vi "Chroma 1905x Series Initialize.vi"(7 "Serial Configuration":T1={"Baud Rate"=9600, "Flow Control"=0, "Parity"=0, "Data Bits"=8, "Stop Bits"=1} {"Flow Control" items=["NONE", "SOFTWARE"]; "Stop Bits" items=["1"=1]; "Data Bits" items=["7"=7, "8"=8]; "Parity" items=["NONE", "ODD", "EVEN"]; "Baud Rate" items=["300"=300, "600"=600, "1200"=1200, "2400"=2400, "4800"=4800, "9600"=9600, "19200"=19200]}, 8 "error in (no error)":errorcluster, 9 "Reset (True)":bool=TRUE, 10 "ID Query (True)":bool=TRUE, 11 "VISA resource name":refnum<visa-resource-name>) -> (0 "error out":errorcluster, 3 "VISA resource name out":refnum<visa-resource-name>)   [LabVIEW 2025]
doc: "This VI passes the addressing information in the instrument decriptor to the Instr Open VI and returns the instrument ID. You can optionally reset the instrument by setting the front panel reset control. You must run this VI before using any of the instrument driver VIs for this instrument."
uses:
  <vilib>/ErrorRing/Error Ring.xnode
  <instrlib>/_Template - Generic/Template - Generic.lvlib
panel:
  # "true\n\nfalse"
  # "true\n\nfalse"
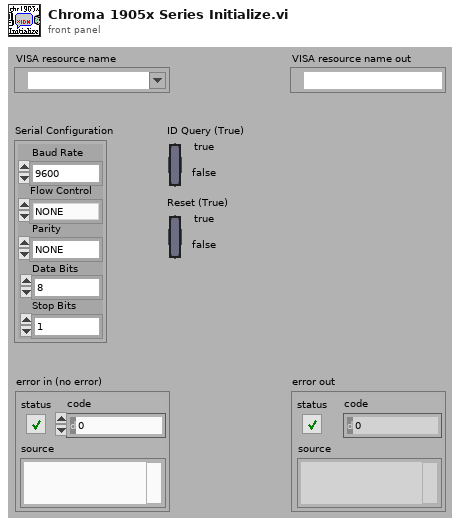
[diagram p1: front panel]
types:
  T1 = cluster{"Baud Rate":u32, "Flow Control":u16, "Parity":u16, "Data Bits":u16, "Stop Bits":u16}
  T2 = cluster{"resource name":string, "interface type":bool, "VISA resource name":refnum<visa-resource-name>}
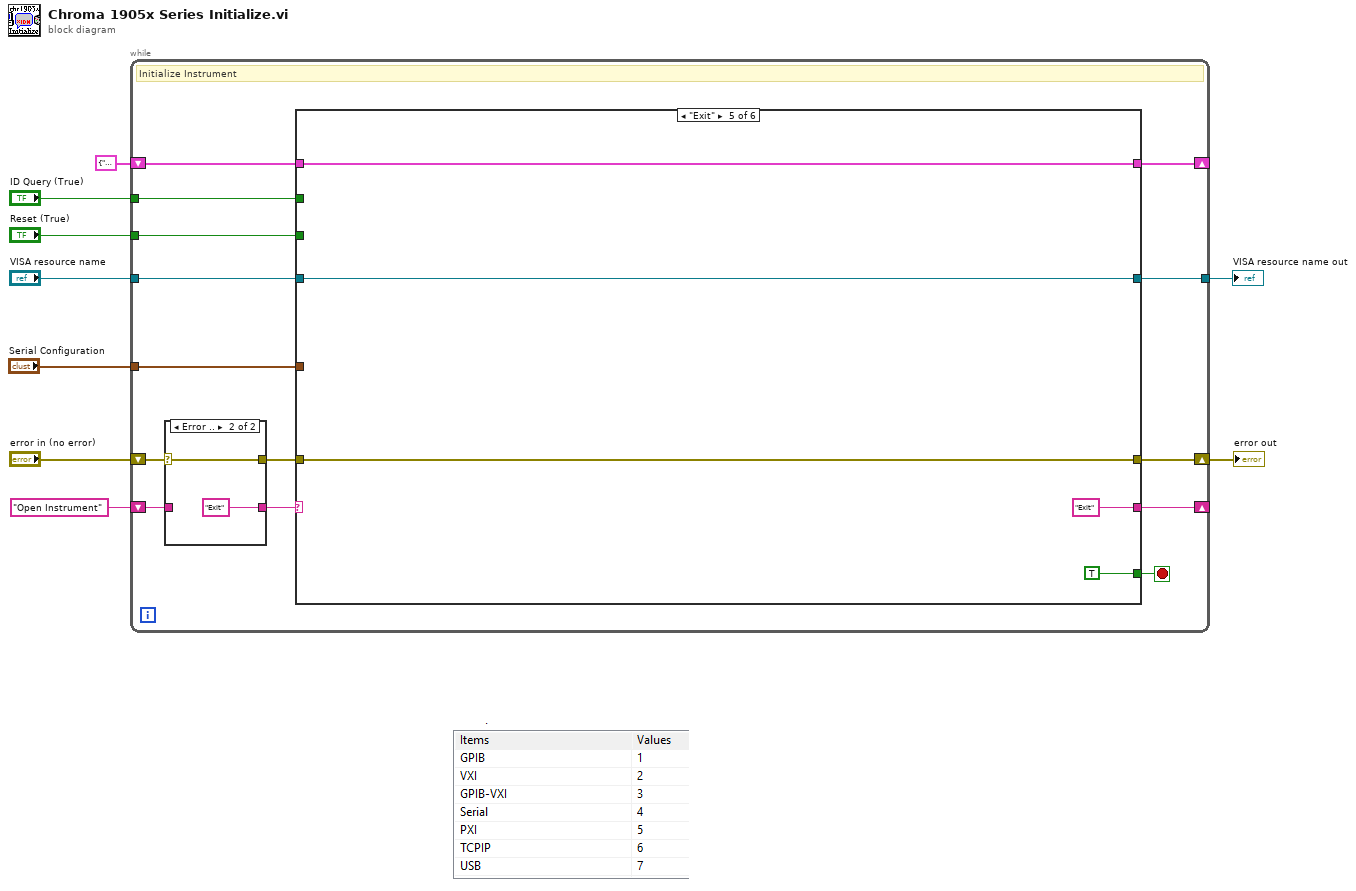
[diagram p0: block diagram]
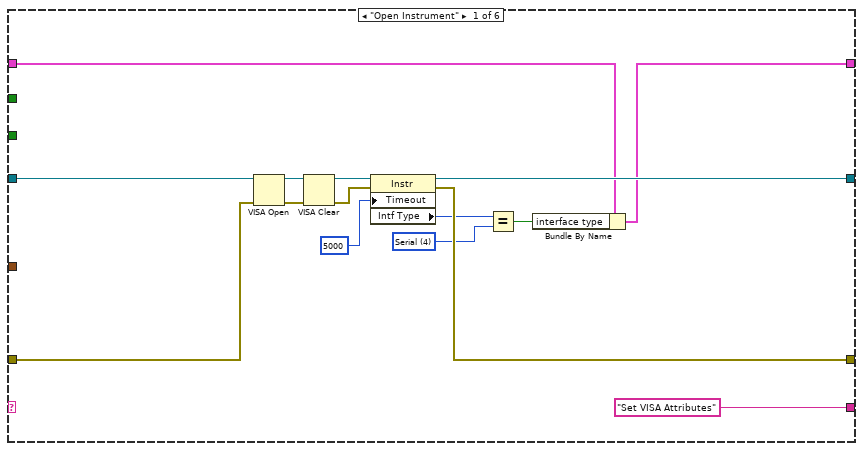
[diagram p3: hidden frame]
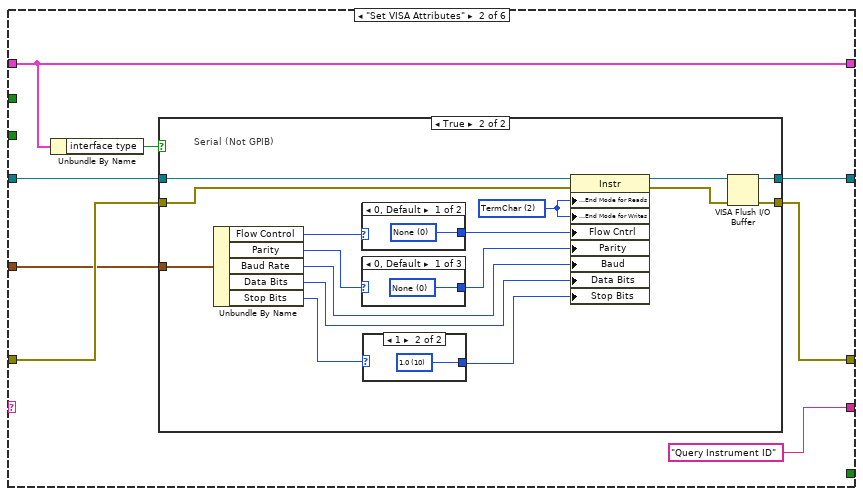
[diagram p4: hidden frame]
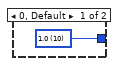
[diagram p6: hidden frame]
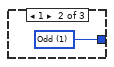
[diagram p7: hidden frame]
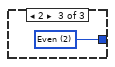
[diagram p8: hidden frame]
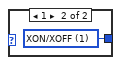
[diagram p9: hidden frame]
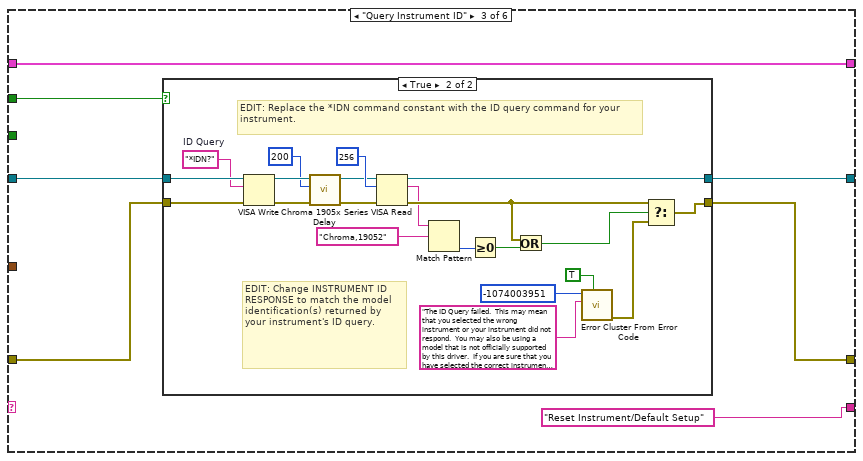
[diagram p10: hidden frame]
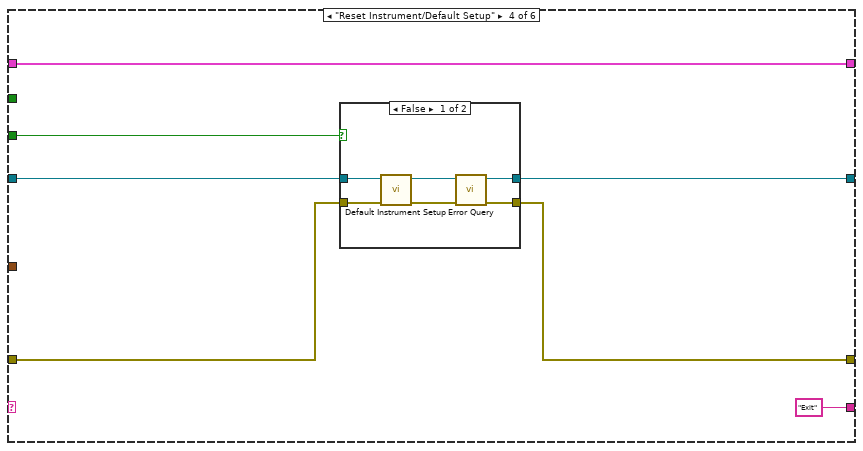
[diagram p12: hidden frame]
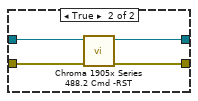
[diagram p13: hidden frame]
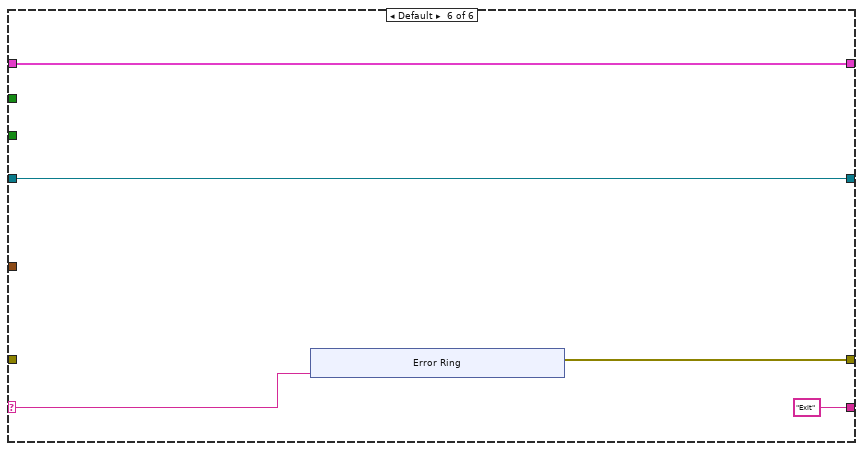
[diagram p14: hidden frame]
diagram:
  n1 = while {
    shift-right: [w22] -> _
    shift-left: T2 {"resource name"="", "interface type"=FALSE, "VISA resource name"=""} -> [w23]
    shift-right: [w21] -> _
    shift-left: "Open Instrument" -> [w14]
    shift-right: [w20] -> w1
    shift-left: "error in (no error)" -> [w16]
    tunnel: [w19] -> w7
    tunnel: "VISA resource name" -> [w18]
    tunnel: "Reset (True)" -> [w12]
    tunnel: "ID Query (True)" -> [w11]
    tunnel: "Serial Configuration" -> [w10]
    stop <- w17 stop-if-true
    # "Initialize Instrument"
    n2 = case shown="Error .." w16 {
      selector: w16 -> [w25 w27]
      tunnel: [w25 w27] -> w15
      tunnel: w14 -> [w24 _]
      tunnel: [w24 "Exit"] -> w13
      frame No Error {
      }
      frame Error {
      }
    }
    n3 = case shown="\"Exit\"" w13 {
      selector: w13 -> [_ _ _ _ _ w130]
      tunnel: w23 -> [w38 w50 w82 w112 w127 w132]
      tunnel: [w37 w50 w82 w112 w127 w132] -> w22
      tunnel: ["Set VISA Attributes" "Query Instrument ID" "Reset Instrument/Default Setup" "Exit" "Exit" "Exit"] -> w21
      tunnel: [w41 w49 w78 w110 w125 w129] -> w20
      tunnel: w15 -> [w39 w47 w80 w111 w125 _]
      tunnel: [w42 w46 w79 w108 w124 w131] -> w19
      tunnel: w18 -> [w32 w44 w81 w109 w124 w131]
      tunnel: [_ _ _ _ TRUE _] -> w17
      tunnel: w12 -> [_ _ _ w106 _ _]
      tunnel: w11 -> [_ _ w76 _ _ _]
      tunnel: w10 -> [_ w43 _ _ _ _]
      frame "Open Instrument" {
        w34 = u16 4 items=["GPIB"=1, "VXI"=2, "GPIB-VXI"=3, "Serial"=4, "PXI"=5] ("Interface Information:Interface Type")
        n4 = VISA Open(error in (no error)=w39, VISA resource name=w32) -> (VISA resource name=w40:refnum<visa-resource-name>, error out=w35:errorcluster)  [unwired: 3 in]
        n5 = VISA Clear(VISA resource name=w40, error in (no error)=w35) -> (VISA resource name out=w31:refnum<visa-resource-name>, error out=w29:errorcluster)
        n6 = property class="Instr"(reference=w31, error in=w29, "Timeout"=u32 5000 ("Tmo Value")) -> (reference out=w42:refnum<visa-resource-name>, error out=w41:errorcluster, "Intf Type"=w30:u16)
        n7 = Equal?(x=w30, y=w34) -> (x = y?=w33:bool)
        n8 = Bundle By Name(cluster=w38, "interface type"=w33) -> (w37:T2)
      }
      frame "Set VISA Attributes" {
        n9 = Unbundle By Name(w50) -> ("interface type"=w48:bool)
        n10 = case shown="True" w48 {
          tunnel: [w51 w64] -> w46
          tunnel: [w52 w65] -> w49
          tunnel: w47 -> [w52 w67]
          tunnel: w44 -> [w51 w68]
          tunnel: w43 -> [_ w54]
          frame False {
            # "GPIB"
          }
          frame True {
            w63 = u16 2 items=["None", "LastBit", "TermChar"] ("Serial Settings:Serial End Mode for Reads")
            # "Serial (Not GPIB)"
            n11 = Unbundle By Name(w54) -> ("Flow Control"=w62:u16, "Parity"=w61:u16, "Baud Rate"=w59:u32, "Data Bits"=w58:u16, "Stop Bits"=w55:u16)
            n12 = case shown="0, Default" w62 {
              tunnel: [w74 w75] -> w57
              frame 0, Default {
                w74 = u16 0 items=["None", "XON/XOFF", "RTS/CTS", "XON/XOFF & RTS/CTS", "DTR/DSR", "XON/XOFF & DTR/DSR"] ("Serial Settings:Flow Control")
              }
              frame 1 {
                w75 = u16 1 items=["None", "XON/XOFF", "RTS/CTS", "XON/XOFF & RTS/CTS", "DTR/DSR", "XON/XOFF & DTR/DSR"] ("Serial Settings:Flow Control")
              }
            }
            n13 = case shown="0, Default" w61 {
              tunnel: [w71 w72 w73] -> w60
              frame 0, Default {
                w71 = u16 0 items=["None", "Odd", "Even", "Mark", "Space"] ("Serial Settings:Parity")
              }
              frame 1 {
                w72 = u16 1 items=["None", "Odd", "Even", "Mark", "Space"] ("Serial Settings:Parity")
              }
              frame 2 {
                w73 = u16 2 items=["None", "Odd", "Even", "Mark", "Space"] ("Serial Settings:Parity")
              }
            }
            n14 = case shown="1" w55 {
              tunnel: [w69 w70] -> w53
              frame 0, Default {
                w69 = u16 10 items=["1.0"=10, "1.5"=15, "2.0"=20] ("Serial Settings:Stop Bits")
              }
              frame 1 {
                w70 = u16 10 items=["1.0"=10, "1.5"=15, "2.0"=20] ("Serial Settings:Stop Bits")
              }
            }
            n15 = property class="Instr"(reference=w68, error in=w67, "Serial Settings:End Mode for Reads"=w63, "Serial Settings:End Mode for Writes"=w63, "Flow Cntrl"=w57, "Parity"=w60, "Baud"=w59, "Data Bits"=w58, "Stop Bits"=w53) -> (reference out=w66:refnum<visa-resource-name>, error out=w56:errorcluster)
            n16 = VISA Flush I/O Buffer(VISA resource name=w66, error in (no error)=w56) -> (VISA resource name out=w64:refnum<visa-resource-name>, error out=w65:errorcluster)  [unwired: 1 in]
          }
        }
      }
      frame "Query Instrument ID" {
        n17 = case shown="True" w76 {
          tunnel: [w83 w105] -> w78
          tunnel: [w84 w102] -> w79
          tunnel: w81 -> [w84 w103]
          tunnel: w80 -> [w83 w104]
          frame False {
          }
          frame True {
            w99 = "*IDN?"  # ID Query
            # "EDIT: Replace the *IDN command constant with the ID query command for your instrument."
            # "EDIT: Change INSTRUMENT ID RESPONSE to match the model identification(s) returned by your instrument's ID query."
            n18 = VISA Write(VISA resource name=w103, write buffer=w99, error in (no error)=w104) -> (VISA resource name out=w89:refnum<visa-resource-name>, error out=w87:errorcluster)  [unwired: 1 out]
            n19 = call "Chroma 1905x Series Delay.vi"("error in (no error)"=w87, "Time Delay [ms]"=u32 200, "VISA resource name"=w89) -> ("error out"=w86:errorcluster, "VISA resource name 2"=w88:refnum<visa-resource-name>)  [unwired: 7 in]
            n20 = VISA Read(VISA resource name=w88, byte count=u32 256, error in (no error)=w86) -> (VISA resource name out=w102:refnum<visa-resource-name>, read buffer=w90:string, error out=w91:errorcluster)  [unwired: 1 out]
            n21 = Match Pattern(string=w90, regular expression="Chroma,19052") -> (offset past match=w94:i32)  [unwired: 1 in, 3 out]
            n22 = Greater Or Equal To 0?(x=w94) -> (x >= 0?=w93:bool)
            n23 = Or(x=w91, y=w93) -> (x .or. y?=w92:bool)
            n24 = call <vilib>:"Error Cluster From Error Code.vi"("show call chain? (False)"=TRUE, "error message (\"\")"="The ID Query failed.  This may mean that you selected the wrong instrument or your instrument did not respond.  You may also be using a model that is not officially supported by this driver.  If you are sure that you have selected the correct instrument and it is responding, try disabling the ID Query." ("Source (VI Name)"), "error code (0)"=-1074003951 ("Code")) -> ("error out"=w98:errorcluster)  [unwired: 6 in]
            n25 = Select(t=w91, s=w92, f=w98) -> (s? t:f=w105:errorcluster)
          }
        }
      }
      frame "Reset Instrument/Default Setup" {
        n26 = case shown="False" w106 {
          tunnel: w111 -> [w118 w122]
          tunnel: [w116 w121] -> w110
          tunnel: w109 -> [w115 w120]
          tunnel: [w113 w119] -> w108
          frame False {
            n27 = call <instrlib>:"Default Instrument Setup.vi"("error in (no error)"=w118, "VISA resource name"=w115) -> ("error out"=w117:errorcluster, "VISA resource name out"=w114:refnum<visa-resource-name>)  [unwired: 8 in]
            n28 = call <instrlib>:"Error Query.vi"("error in (no error)"=w117, "VISA resource name"=w114) -> ("error out"=w116:errorcluster, "VISA resource name out"=w113:refnum<visa-resource-name>)  [unwired: 6 in, 2 out]
          }
          frame True {
            n29 = call "Chroma 1905x Series 488.2 Cmd -RST.vi"("error in (no error)"=w122, "VISA resource name"=w120) -> ("error out"=w121:errorcluster, "VISA resource name out"=w119:refnum<visa-resource-name>)  [unwired: 8 in]
          }
        }
      }
      frame "Exit" {
      }
      frame Default {
        n30 = xnode "Error Ring"("parameter 0"=w130) -> ("error out"=w129:errorcluster)
      }
    }
  }
  "VISA resource name out" <- w7
  "error out" <- w1
